vi "MHM FullAcquisition.vi"(8 "error in (no error)":errorcluster, 10 "ulCycles":u32, 11 "ulMHMHandle":u32) -> (0 "error out":errorcluster, 3 "function return":u32)   [LabVIEW 2017, in "MHM_1SL_interface.lvlib"]
uses:
  MHM_1SL_interface.lvlib
  lib/MHM_1SL_interface.dll
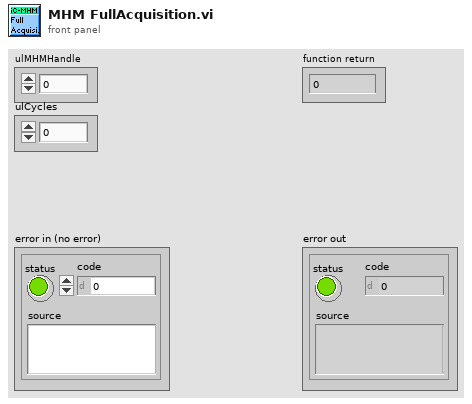
[diagram p1: front panel]
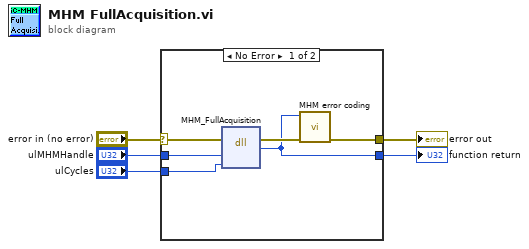
[diagram p0: block diagram]
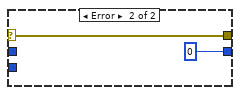
[diagram p2: hidden frame]
diagram:
  n1 = case shown="No Error" "error in (no error)" {
    selector: "error in (no error)" -> [w11 w13]
    tunnel: "ulMHMHandle" -> [w10 _]
    tunnel: [w8 w13] -> w3
    tunnel: [w7 u32 0] -> w2
    tunnel: "ulCycles" -> [w6 _]
    frame No Error {
      n2 = dll-call lib="C:/workspace/project/scancon/sw/SSI_Tool/DUT_Interface/lv_interface/lib/MHM_1SL_interface.dll" fn="MHM_FullAcquisition"(error in=w11, "ulMHMHandle"=w10, "ulCycles"=w6) -> (error out=w9:errorcluster, "return type"=w7:u32)  [unwired: 4 in, 1 out]
      n3 = call "MHM error coding.vi"("error in (no error)"=w9, "function return in"=w7) -> ("error out"=w8:errorcluster)  [unwired: 9 in]
    }
    frame Error {
    }
  }
  "function return" <- w2
  "error out" <- w3
